vi "Function Generator.vi"() -> ()   [LabVIEW 2020]
uses:
  <vilib>/measure/NI_MABase.lvlib
panel:
  in  "signal type":T1(ring)
  out "Waveform Graph":waveform(dbl)(graph)
  in  "stop":bool
  in  "Phase":dbl
  in  "Frequency":dbl(knob) scale=0.0..100.0
  in  "Amplitude":dbl(knob) scale=0.0..10.0
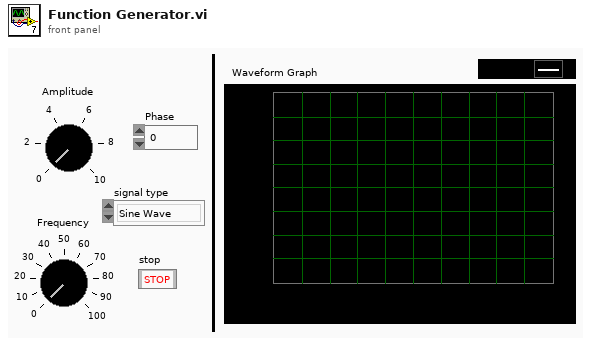
[diagram p1: front panel]
types:
  T1 = enum16{"Sine Wave", "Triangle Wave", "Square Wave", "Sawtooth Wave"}
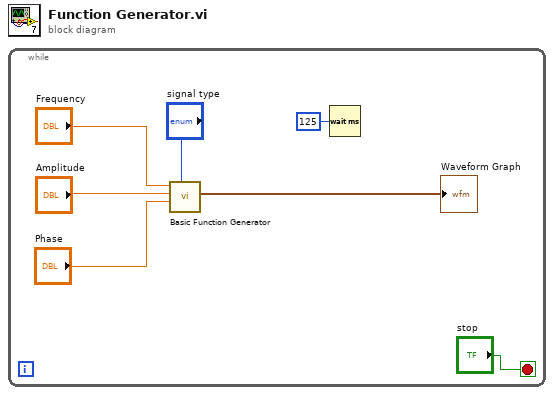
[diagram p0: block diagram]
diagram:
  n1 = while {
    stop <- "stop" stop-if-true
    n2 = call <vilib>:"Basic Function Generator.vi"("signal type"="signal type", "phase"="Phase", "amplitude"="Amplitude", "frequency"="Frequency") -> ("signal out"=→"Waveform Graph":waveform(dbl))  [unwired: 5 in, 2 out]
    n3 = Wait (ms)(milliseconds to wait=u32 125) -> ()  [unwired: 1 out]
  }
